vi "PLC.ReadPLCData.vi"(7 "Idx":i32, 8 "error in (no error)":errorcluster, 9 "Sets":T2, 10 "PLCdata in":T3, 11 "Ref in":u64) -> (0 "error out":errorcluster, 1 "Events":T1[](array[typedef]), 2 "PLCdata out":T3, 3 "Ref out":u64)   [LabVIEW 2016]
doc: "Read data block from PLC to PC, check live bit of PLC\n\nWabco 2017 All right reserved\nAuthor: maciej.szupienko@wabco-auto.com"
uses:
  PLC.DataBlock.PLCstatus.ctl
  PLC.DataBlock.PLCstatus.General.ctl
  PLC.DataBlock.PLCstatus.Station.ctl
  PLC.Data.Sets.ctl
  tools/EventLog/EventLog.EventSource.ctl
  tools/EventLog/EventLog.CreateError(array).vi
  tools/Translator/Translator.Translate.Status (NoError).vi
  tools/Translator/Translator.FormatMessage.vi
  tools/Translator/Translator.Global.vi
  tools/ErrorHandling/ErrorHandling.Create.vi
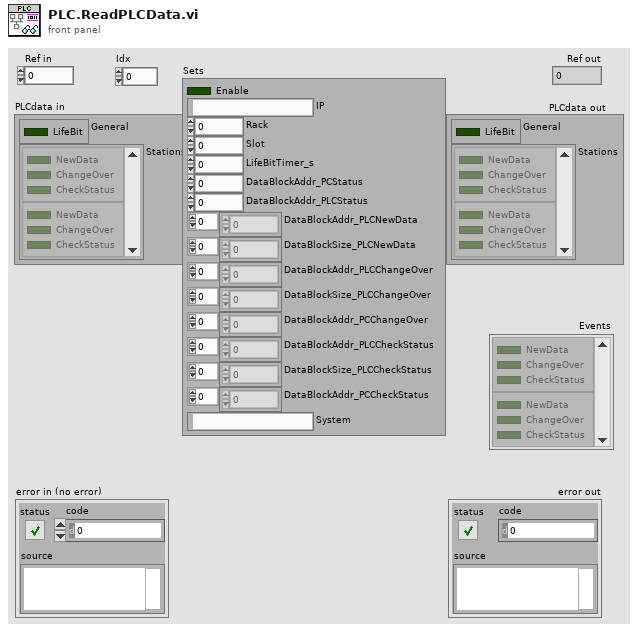
[diagram p1: front panel]
types:
  T1 = typedef "PLC.DataBlock.PLCstatus.Station.ctl" = cluster{"NewData":bool, "ChangeOver":bool, "CheckStatus":bool}
  T2 = typedef "PLC.Data.Sets.ctl" = cluster{"Enable":bool, "IP":string, "Rack":i32, "Slot":i32, "LifeBitTimer_s":dbl, "DataBlockAddr_PCStatus":i32, "DataBlockAddr_PLCStatus":i32, "DataBlockAddr_PLCNewData":i32[], "DataBlockSize_PLCNewData":i32[], "DataBlockAddr_PLCChangeOver":i32[], "DataBlockSize_PLCChangeOver":i32[], "DataBlockAddr_PCChangeOver":i32[], "DataBlockAddr_PLCCheckStatus":i32[], "DataBlockSize_PLCCheckStatus":i32[], "DataBlockAddr_PCCheckStatus":i32[], "System":string}
  T3 = typedef "PLC.DataBlock.PLCstatus.ctl" = cluster{"General":T4, "Stations":T1[]}
  T4 = typedef "PLC.DataBlock.PLCstatus.General.ctl" = cluster{"LifeBit":bool}
  T5 = typedef "EventLog.EventSource.ctl" = enum16{"All", "Gui", "Ref", "File", "Arch", "Seq", "CPX", "DB", "Laser", "Scan.P", "Scan.O", "PLC"}
  T6 = enum16{"-", "Event confirmed", "Log out", "Log in", "Shutdown", "Cancel", "Start", "Begin time", "End time", "Duration", "Service Mode", "Ignore Results", "Serial Format", "On", "Off", "OK", "NOK", "NOK %s", "Home", "Work", "Close", "Open", "In progress...", "Missing", "Empty", "Hardware failure", "Initial", "Default", "Total", "Out of range", "Free disk space is below 1GB - contact technician", "Error %d >> %s", "Error %d >> %s >> %s", "Msg %d >> %s", "Laser msg %d %s", "Laser cmd error %s %d", "Laser cmd failed %s", "Laser cmd warning %s", "Laser disconnected", "Laser status %s", "Laser already started", "Laser job unkonwn %s", "Laser job missing %s", "Laser job select failure %s", "Unable to start laser printing (%s)", "Unable to stop laser printing (%s)", "Laser marking aborted", "Laser marking timeout", "Unable to reset Laser Interlock (%s)", "Unable to trigger Laser. Laser not ready (%s)", "Laser job '%s' coordinates not configured", "Starting %s", "Quitting %s", "Configured", "Initializing", "Quitting", "Loading", "Loaded %d results", "Loaded %d events", "Running", "Stopped", "Summary", "Laser", "Do you want to continue?", "Do you want to delete the configuration?", "The configuration is being used by an order. Unable to delete!", "Press confirm button", "Station is not based. Do you want to exit?", "Station requires changeover. Do you want to run the test?", "Test options are not set as default. Do you want to continue?", "Formatting of WabcoNo is disabled. Do you want to continue?", "Product not detected. Do you want to continue?", "Product scan failed. Do you want to continue?", "Calibration", "Log out?", "System", "All", "IDLE", "Translating...%s", "Not found", "Alarm %s", "Run", "Skip", "Abort", "Repeat", "Please wait...", "Database disconnected", "Database disconnected - changeover disabled!", "Login to database successful", "Login to database failed: %d; %s", "Unable to check the product status of reference %d - database disconnected", "Unable to set the product status of reference %d - database disconnected", "Variant file backup %s", "Read variant (%s)", "Result", "Station armed!", "Station requires changeover!", "Select reference number...", "EMERGENCY BUTTON - press Control button", "EMERGENCY DOOR - press Control button", "Resetting Emergency...", "Unable to reset safety circuit - Emergency Button pressed", "Unable to reset safety circuit - Emergency Side Door open", "Station not based", "Station based", "Station not empty", "Station basing...", "No order", "Press Start to begin new order", "Scanning new order", "Order NOK. Correct or scan again", "Order OK. Press Accept", "Order ready", "Revolver incorrect", "Fork incorrect", "Revolver missing", "Revolver empty", "Container missing", "Offline results", "Offline statistics", "Updating statistics %.1f %%", "DMC Configurator", "Door open", "Close the front door", "Press start button", "Done. Open the front door", "Running...", "Running...%.1f %%", "Pause %s", "Pause %s. NOK container missing", "Pause %s. OK container missing", "Pause %s. Revolver empty", "Pause %s. Revolver missing", "Pause %s. Revolver incorrect", "Pause %s. Fork missing", "Pause %s. Fork incorrect", "Pause %s. Too many failures", "Pause %s. Unloading failure", "Pause %s. One slot is not working", "Pause %s. Part order is done. Empty OK container", "Pause %s. Unable to move product to slot", "Pause %s. Unable to move back product pusher", "Pause %s. Unable to lift product", "Pause %s. Unable to move back product lifter", "Pause %s. Unable to move product arm to Work", "Pause %s. Unable to move product arm to NOK", "Pause %s. Unable to move product arm to OK", "Pause %s. Unable to unsuck the NOK product", "Pause %s. Unable to drop the NOK product", "Pause %s. Product OK missing", "Pause %s. Unable to unsuck the OK product", "Pause %s. Unable to drop the OK product", "Stopping...", "File '%s' is missing", "File '%s' is broken", "File '%s' is running", "Log file started (%s)", "Log file ended (%s)", "Log file stopped (%s)", "Log file ignored (%s)", "Log file exported (%s)", "Log file export failed (%s)", "Wrong serial number in log file", "Wrong reference number in log file", "Test steps are missing", "%s = %.3f", "Process param '%s' not found in DB", "Process param '%s' wrong order", "Process param '%s' value %.3f out of limits (%.3f; %.3f)", "Step%d param '%s' not found in DB", "Step%d param '%s' wrong order", "Step%d param '%s' value %.3f out of limits (%.3f; %.3f)", "Step%d EV '%s' not found in DB", "Step%d EV '%s' wrong order", "\"%s\" not found in DB", "\"%s\" wrong order", "\"%s\" value %.3f out of limits (%.3f; %.3f)", "\"%s\" not found in software", "Process init (%s)", "Process started", "Process restarted", "Process run", "Process done", "Process done - remove OK container", "Process aborted", "Process aborted at work", "Process aborted at home", "Process error", "Process error at home", "Process error at work", "Process close", "Process pause", "Process continue", "Process door open", "Process door close", "Process pause at slot %s due to %s", "Select plate from the order to process", "Do you want to start the process?", "Do you want to continue the process?", "There is unfinished order. Do you want to put the new order?", "Product %s %d OK", "Product %s %d NOK", "Unable to unload the slot %s. Product missing in the slot", "Unable to unload the slot %s. Product already in the arm", "Unable to accept the product as OK. Product missing in slot %s", "Unable to accept the product as OK. Product could not drop into the container at slot %s", "Unable to accept the product as NOK. Product could not drop into the container at slot %s", "Scan failed. Error %s", "Scan failed. Scanner disconnected", "Scan failed. Wrong Wabco number %d, limit (%d,%d)", "Scan failed. Wrong serial number %d, limit (%d,%d)", "Scan failed. Wrong date %d, limit (%d,%d)", "Scan failed. Wrong product wabco number %d (expected %d)", "Scan failed. Wrong product serial number %d (expected > 0)", "Scan OK %s", "Scan failed. Unable to determine table position (%s)", "Scan failed. Timeout", "Tune failed. Scanner disconnected", "Tune failed. Timeout", "%s = %d", "%s = %d->%d", "Unable to set %s = %.2f - Air Pressure Inside off", "Unable to set digital output '%s' = %d", "Unable to activate air pressure inside - timeout", "Unable to activate air pressure inside - aborted", "Unable to switch on Air Main Valve - Air Pressure Inlet off", "Unable to switch on Air Main Valve - Door open", "Unable to switch off Air Main Valve - timeout", "Unable to switch off Air Main Valve - aborted", "Unable to rotate Table - timeout", "Unable to rotate Table - aborted", "Unable to rotate Table - Product Move not in Home position", "Unable to rotate Table - Air Pressure Inside off", "Unable to rotate Table - Product Lift A not in Home position", "Unable to rotate Table - Product Lift B not in Home position", "Unable to rotate Table - unlock before movement timeout", "Unable to rotate Table - lock after movement timeout", "Unable to move Table Lock to %s position - timeout", "Unable to move Table Lock to %s position - aborted", "Unable to move Table Lock to %s position - Air Pressure Inside off", "Unable to move Table Lock to %s position - Table not in position", "Unable to move Product Lift A to %s position - timeout", "Unable to move Product Lift B to %s position - timeout", "Unable to move Product Lift A to %s position - aborted", "Unable to move Product Lift B to %s position - aborted", "Unable to move Product Lift A to %s position - Air Pressure Inside off", "Unable to move Product Lift B to %s position - Air Pressure Inside off", "Unable to move Product Lift A to %s position - Table not locked", "Unable to move Product Lift B to %s position - Table not locked", "Unable to move Product Lift A to %s position - Product Arm not in Work position", "Unable to move Product Lift B to %s position - Product Arm not in Work position", "Unable to set Product Suction Gripper %s to %s - timeout", "Unable to set Product Suction Gripper %s to %s - aborted", "Unable to set Product Suction Gripper %s to %s - Air Pressure Inside off", "Unable to set Product Suction Gripper %s to %s - Table slot unkown", "Unable to move Product Arm to %s position - timeout", "Unable to move Product Arm to %s position - aborted", "Unable to move Product Arm to %s position - Air Pressure Inside off", "Unable to move Product Arm to %s position - Product Lift A not in Home position", "Unable to move Product Arm to %s position - Product Lift B not in Home position", "Unable to move Product to %s position - timeout", "Unable to move Product to %s position - aborted", "Unable to move Product to %s position - Air Pressure Inside off", "Unable to move Product to %s position - Table not in position"}
  T7 = cluster{"Boolean array[0]":bool, "Boolean array[1]":bool, "Boolean array[2]":bool, "Boolean array[3]":bool, "Boolean array[4]":bool, "Boolean array[5]":bool, "Boolean array[6]":bool, "Boolean array[7]":bool}
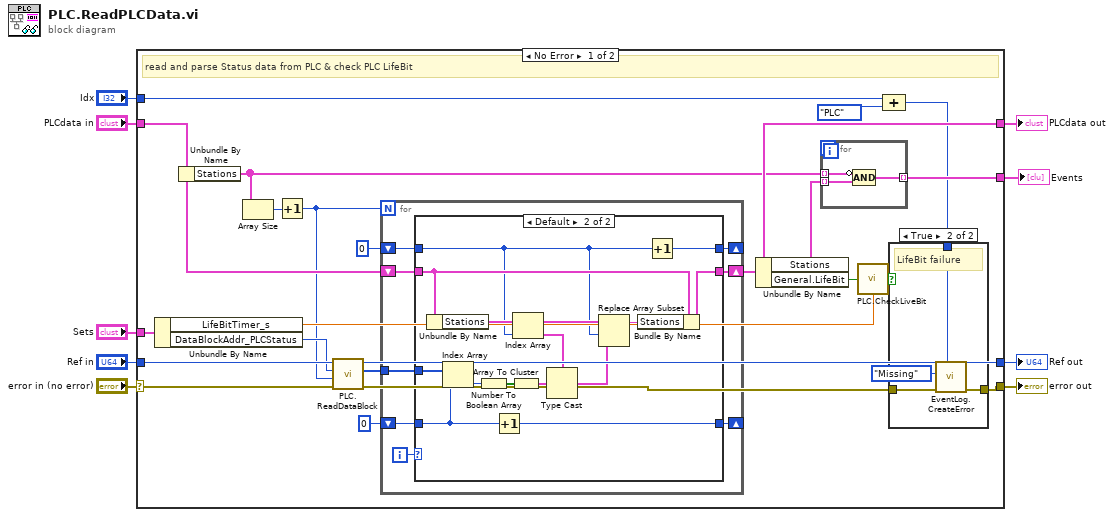
[diagram p0: block diagram]
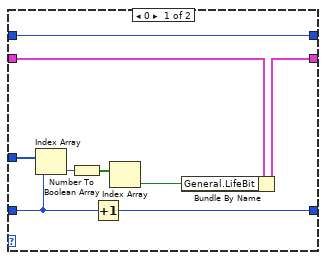
[diagram p2: hidden frame]
diagram:
  n1 = case shown="No Error" "error in (no error)" {
    selector: "error in (no error)" -> [w30 w74]
    tunnel: "Ref in" -> [w32 w73]
    tunnel: [w25 w74] -> w8
    tunnel: "PLCdata in" -> [w21 w72]
    tunnel: [w19 w72] -> w6
    tunnel: [w31 w73] -> w5
    tunnel: "Sets" -> [w29 _]
    tunnel: [w18 _] -> w1
    tunnel: "Idx" -> [w13 _]
    frame No Error {
      # "read and parse Status data from PLC & check PLC LifeBit"
      n2 = Unbundle By Name(w29) -> ("LifeBitTimer_s"=w24:dbl, "DataBlockAddr_PLCStatus"=w28:i32)
      n3 = Unbundle By Name(w21) -> ("Stations"=w17:T1[])
      n4 = Array Size(array=w17) -> (size(s)=w15:i32)
      n5 = Increment(x=w15) -> (x+1=w14:i32)
      n6 = call "PLC.ReadDataBlock.vi"("error in (no error)"=w30, "Amount (1)"=w14, "Block"=w28, "Ref"=w32) -> ("error out"=w26:errorcluster, "data out"=w23:u8[], "ref out"=w31:u64)  [unwired: 5 in]
      n7 = for {
        N: w14 -> [_]
        tunnel: w23 -> [w35]
        shift-right: [w38] -> _
        shift-left: 0 -> [w39]
        shift-right: [w36] -> w19
        shift-left: w21 -> [w37]
        shift-right: [w33] -> _
        shift-left: 0 -> [w34]
        i -> [w40]
        n8 = case shown="Default" w40 {
          tunnel: w39 -> [w42 w50]
          tunnel: [w46 w60] -> w38
          tunnel: w37 -> [w49 w59]
          tunnel: [w45 w62] -> w36
          tunnel: w35 -> [w48 w63]
          tunnel: w34 -> [w41 w51]
          tunnel: [w41 w52] -> w33
          frame 0 {
            n9 = Index Array(array=w48, index=w42) -> (element=w47:u8)
            n10 = Number To Boolean Array(number=w47) -> (Boolean array=w44:bool[])
            n11 = Increment(x=w42) -> (x+1=w46:i32)
            n12 = Index Array(array=w44) -> (element=w43:bool)  [unwired: 1 in]
            n13 = Bundle By Name(cluster=w49, "General.LifeBit"=w43) -> (w45:T3)
          }
          frame Default {
            n14 = Unbundle By Name(w59) -> ("Stations"=w55:T1[])
            n15 = Index Array(array=w63, index=w50) -> (element=w61:u8)
            n16 = Number To Boolean Array(number=w61) -> (Boolean array=w57:bool[])
            n17 = Increment(x=w50) -> (x+1=w60:i32)
            n18 = Array To Cluster(array=w57) -> (cluster=w56:T7)
            n19 = Index Array(array=w55, index=w51) -> (element=w54:T1)
            n20 = Type Cast(type=w54, x=w56) -> (*(type *) &x=w53:T1)
            n21 = Replace Array Subset(array=w55, new element=w53, index=w51) -> (w58:T1[])
            n22 = Bundle By Name(cluster=w59, "Stations"=w58) -> (w62:T3)
            n23 = Increment(x=w51) -> (x+1=w52:i32)
          }
        }
      }
      n24 = Unbundle By Name(w19) -> ("Stations"=w16:T1[], "General.LifeBit"=w20:bool)
      n25 = for {
        tunnel: w17 -> [w65] mode=indexing
        tunnel: w16 -> [w64] mode=indexing
        tunnel: [w66] -> w18 mode=indexing
        n26 = Compound Arithmetic op=AND(invert w65, w64) -> (w66:T1)
      }
      n27 = call "PLC.CheckLiveBit.vi"("LifeBit"=w20, "Timer [s] (3)"=w24) -> ("LiveBitElapsed"=w27:bool)
      n28 = Compound Arithmetic op=ADD(w13, EventLog.EventSource."PLC" ("Event source")) -> (w12:i32)
      n29 = case shown="True" w27 {
        tunnel: w26 -> [w67 w71]
        tunnel: [w67 w70] -> w25
        tunnel: w12 -> [_ w69]
        frame False {
        }
        frame True {
          # "LifeBit failure"
          n30 = call-poly "EventLog.CreateError.vi"("Source (All)"=w69, "error in"=w71, "msg"=T6."Missing") -> ("error out"=w70:errorcluster)  [unwired: 7 in, 1 out]
        }
      }
    }
    frame Error {
    }
  }
  "PLCdata out" <- w6
  "error out" <- w8
  "Ref out" <- w5
  "Events" <- w1
